vi "Lookup Local Channels.vi"(6 "VolatusAPI":refnum<class "VolatusAPI.lvclass">, 8 "error in (no error)":errorcluster, 11 "LocalGraphBuffer in":refnum<class "LocalGraphBuffer.lvclass">) -> (0 "error out":errorcluster, 2 "Has Local":bool, 3 "LocalGraphBuffer out":refnum<class "LocalGraphBuffer.lvclass">)   [LabVIEW 2020, in "VolatusGUIElements.lvlib" / "LocalGraphBuffer.lvclass"]
uses:
  LocalGraphBuffer.lvclass
  Volatus/VolatusAPI/VolatusAPI.lvclass
  Volatus/VolatusAPI/VolatusAPI.lvclass/VolatusAPI.ctl
  LocalGraphBuffer.lvclass/LocalGraphBuffer.ctl
  lv-vecto/Vecto/Channel DBL/Channel DBL.lvclass/Channel DBL.ctl
  lv-vecto/Vecto/Group DBL/Group DBL.lvclass
  C:/dev/lv20CE/relink/lv-vecto/Vecto/Group/Group.lvclass
  lv-vecto/Vecto/ChannelService/Lookup Double Channel.vi
  lv-vecto/Vecto/Group/Channel Info by Index.vi
  lv-vecto/Vecto/Channel DBL/Channel DBL.lvclass
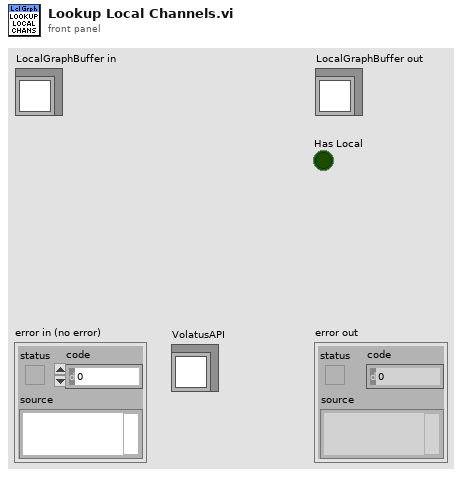
[diagram p1: front panel]
types:
  T1 = typedef "VolatusGUIElements.lvlib/LocalGraphBuffer.lvclass/Plot.ctl" = cluster{"Data Q":refnum<queue>, "Time Q":refnum<queue>, "Group":string, "Channel Index":i32, "Local":bool, "Channel":refnum<class "Channel DBL.lvclass">}
  T2 = typedef "VectoConfig.lvlib/Channel Info.ctl" = cluster{"Name":string, "Group":string, "Owning Node":string, "Owning Task":string, "Resource":string}
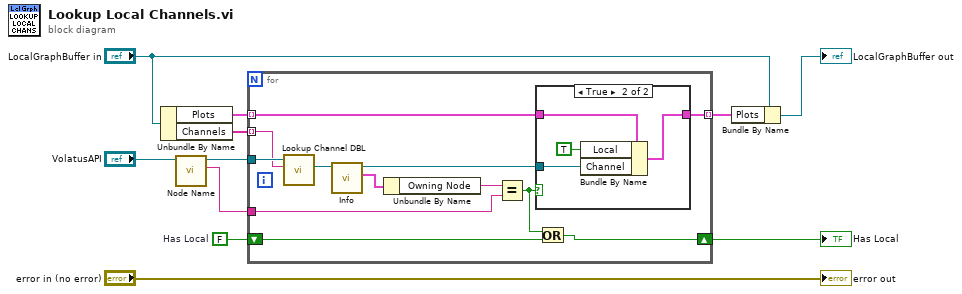
[diagram p0: block diagram]
diagram:
  w2 = FALSE  # Has Local
  n1 = Unbundle By Name("LocalGraphBuffer in") -> ("Plots"=w5:T1[], "Channels"=w9:string[])
  n2 = call "Node Name.vi"("VolatusAPI in"="VolatusAPI") -> ("Node Name"=w6:string, "VolatusAPI out"=w7:refnum<class "VolatusAPI.lvclass">)  [unwired: 8 in, 1 out]
  n3 = for {
    tunnel: w9 -> [w12] mode=indexing
    tunnel: w7 -> [w23]
    tunnel: w6 -> [w19]
    tunnel: w5 -> [w18] mode=indexing
    tunnel: [w16] -> w3 mode=indexing
    shift-right: [w13] -> w1
    shift-left: w2 -> [w15]
    n4 = call "Lookup Channel DBL.vi"("Name"=w12, "VolatusAPI in"=w23) -> ("Channel DBL"=w22:refnum<class "Channel DBL.lvclass">)  [unwired: 7 in, 2 out]
    n5 = call "Info.vi"("Channel in"=w22) -> ("Info"=w21:T2, "Channel out"=w17:refnum<class "Channel DBL.lvclass">)  [unwired: 8 in, 1 out]
    n6 = Unbundle By Name(w21) -> ("Owning Node"=w20:string)
    n7 = Equal?(x=w20, y=w19) -> (x = y?=w14:bool)
    n8 = case shown="True" w14 {
      tunnel: w18 -> [w24 w28]
      tunnel: w17 -> [_ w27]
      tunnel: [w24 w26] -> w16
      frame False {
      }
      frame True {
        n9 = Bundle By Name(cluster=w28, "Local"=TRUE, "Channel"=w27) -> (w26:T1)
      }
    }
    n10 = Or(x=w14, y=w15) -> (x .or. y?=w13:bool)
  }
  "Has Local" <- w1
  n11 = Bundle By Name(cluster="LocalGraphBuffer in", "Plots"=w3) -> (→"LocalGraphBuffer out":refnum<class "LocalGraphBuffer.lvclass">)
  "error out" <- "error in (no error)"
